vi "Read Measurement.vi"(6 "Enable Relative Mode (F: Disable)":bool, 7 "Combination (0: Single)":dbl(ring) items=["Single", "Feed1-Feed2", "Feed1/Feed2"], 8 "error in (no error)":errorcluster, 9 "Measurement Number (0: <0>)":i32(ring) items=["Measurement 1"=1, "Measurement 2"=2, "Measurement 3"=3, "Measurement 4"=4], 10 "Maximum Time (30000 ms)":dbl=30000.0, 11 "VISA resource name":refnum<visa-resource-name>) -> (0 "error out":errorcluster, 2 "Measurement Data (dBm or Volt)":dbl, 3 "VISA resource name out":refnum<visa-resource-name>)   [LabVIEW 2011, in "Agilent N432A.lvlib"]
doc: "Reads the measurement data depending on the combination and relative mode settings. The combination parameter must be the same as that configured in the Configure Measurement.vi and the relative mode parameter must be the same as that configured in the Configure Relative Measurement.vi.\n\n<B>Note:</B>\n\nYou must use the Configure Measurement.vi and Configure Relative Measurement.vi to set the power meter before using this VI to read data."
uses:
  <instrlib>/Agilent N432A/Agilent N432A.lvlib
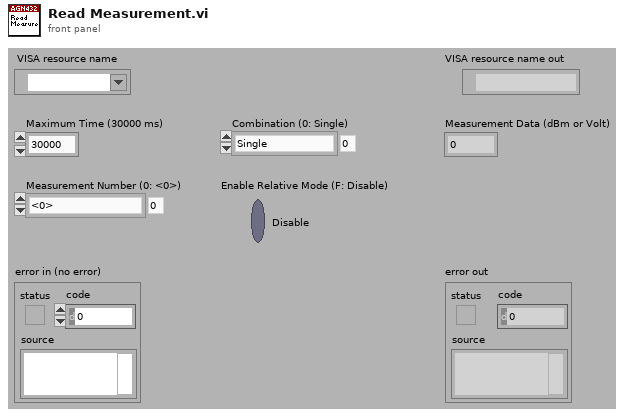
[diagram p1: front panel]
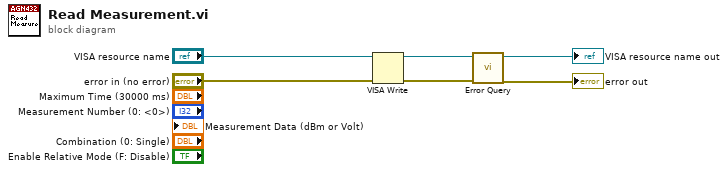
[diagram p0: block diagram]
diagram:
  n1 = VISA Write(VISA resource name="VISA resource name", error in (no error)="error in (no error)") -> (VISA resource name out=w4:refnum<visa-resource-name>, error out=w3:errorcluster)  [unwired: 1 in, 1 out]
  n2 = call <instrlib>:"Error Query.vi"("error in (no error)"=w3, "VISA resource name"=w4) -> ("error out"=→"error out":errorcluster, "VISA resource name out"=→"VISA resource name out":refnum<visa-resource-name>)  [unwired: 6 in, 2 out]
